vi "New (Array).vi"(8 "error in (no error)":errorcluster, 9 "aggregation method (all)":T2=enum."All", 10 "match behavior (keep)":T1, 11 "regex strings":string[](array[string])) -> (0 "error out":errorcluster, 3 "regex out":refnum<class "Regex.lvclass">)   [LabVIEW 2018, in "Logging.lvlib" / "Regex.lvclass"]
uses:
  Regex.lvclass
  C:/Users/Colin/Documents/software_projects/glog/Logging/Filters/Filter/Filter.lvclass
  Aggregation Method.ctl
  Match Behavior.ctl
  Regex.lvclass/Regex.ctl
  Filter/Filter.lvclass/Filter.ctl
  <vilib>/regexp/Match Regular Expression.xnode
  Filter/Filter.lvclass
  Logging.lvlib
panel:
  # "Connector Pane"
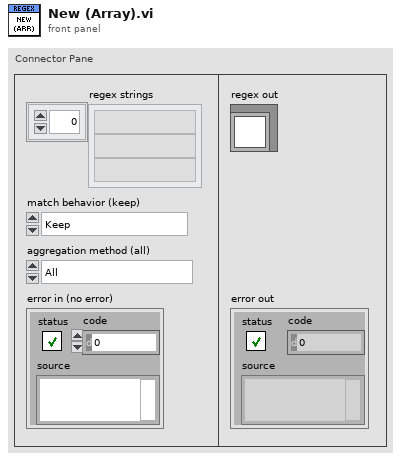
[diagram p1: front panel]
types:
  T1 = typedef "Logging.lvlib/Match Behavior.ctl" = enum16{"Keep", "Discard"}
  T2 = typedef "Logging.lvlib/Aggregation Method.ctl" = enum16{"Any", "Only", "All", "None"}
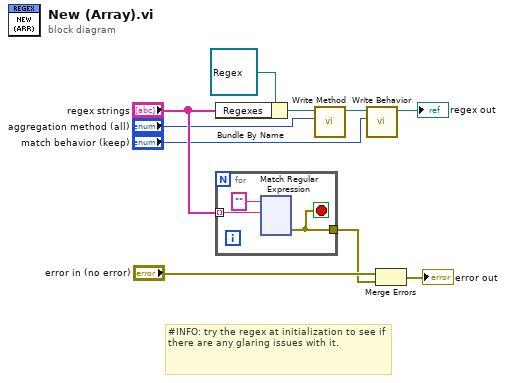
[diagram p0: block diagram]
diagram:
  # "#INFO: try the regex at initialization to see if there are any glaring issues with it."
  n1 = Bundle By Name(cluster=refnum<class "Regex.lvclass"> refnum ("Regex in"), "Regexes"="regex strings") -> (w9:refnum<class "Regex.lvclass">)
  n2 = for {
    tunnel: [w11] -> w7
    tunnel: "regex strings" -> [w12] mode=indexing
    stop <- w11 stop-if-true
    n3 = xnode "Match Regular Expression"("input string"="", "regular expression"=w12) -> ("error out"=w11:errorcluster)  [unwired: 4 in, 4 out]
  }
  n4 = call "Write Method.vi"("Method"="aggregation method (all)", "Filter in"=w9) -> ("Filter out"=w4:refnum<class "Regex.lvclass">)  [unwired: 9 in]
  n5 = call "Write Behavior.vi"("match behavior"="match behavior (keep)", "Filter in"=w4) -> ("Filter out"=→"regex out":refnum<class "Regex.lvclass">)  [unwired: 9 in]
  n6 = Merge Errors("error in (no error)", w7) -> (→"error out":errorcluster)
